vi "PCO_Init.vi"() -> (0 "ErrorOut":errorcluster, 2 "BufferID":i16[](array[numeric]), 3 "hout":u64, 4 "SizeVer":u16, 5 "Bits/pixel":u16, 6 "SizeHor":u16, 8 "PixelRates":u32[](array[numeric]))   [LabVIEW 2014]
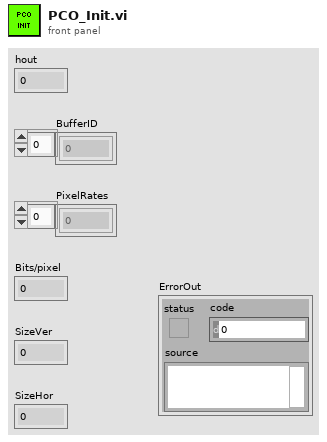
[diagram p1: front panel]
types:
  T1 = cluster{"Size":u16, "SensorTypeDESC":u16, "SensorSubtypeDESC":u16, "MaxHorizontalResStdDESC":u16, "MaxVerticalResStdDESC":u16, "MaxHorizontalResExtDESC":u16, "MaxVerticalResExtDESC":u16, "DynResDESC":u16, "MaxBinHorzDESC":u16, "BinHorzStepDESC":bool, "MaxBinVertDESC":u16, "BinVertStepDESC":bool, "ROIHorzStepDESC":u16, "ROIVertStepDESC":u16, "NumADCDESC":u16, "IRDESC":bool, "MinDelayDESC":u32, "MaxDelayDESC":u32, "MinDelayStepDESC":u32, "MinExpoDESC":u32, "MaxExpoDESC":u32, "MinExpoStepDESC":u32, "MinDelayIRDESC":u32, "MaxDelayIRDESC":u32, "MinExpoIRDESC":u32, "MaxExpoIRDESC":u32, "TimeTableDESC":bool, "DoubleImageDESC":bool, "MinCoolSetDESC":i16, "MaxCoolSetDESC":i16, "MDefaultCoolSetDESC":i16, "PowerDownModeDESC":bool, "OffsetRegDESC":bool, "ColorPattern":cluster{"UpperLeftColor":u8, "UpperRightColor":u8, "LowerLeftColor":u8, "LowerRightColor":u8}, "PatternTypeDESC":bool, "PixelRates":u32[], "CoversionFactors":u16[], "Reserved":u32[], "NoiseFilterCapable":bool, "HotPixelCapable":bool, "HotPixelWithNoiseFilter":bool, "ASCIITimeCapable":bool, "Extended Description":bool, "Get Extended":bool, "Reserved Flag 1":bool, "Reserved Flag 2":bool}
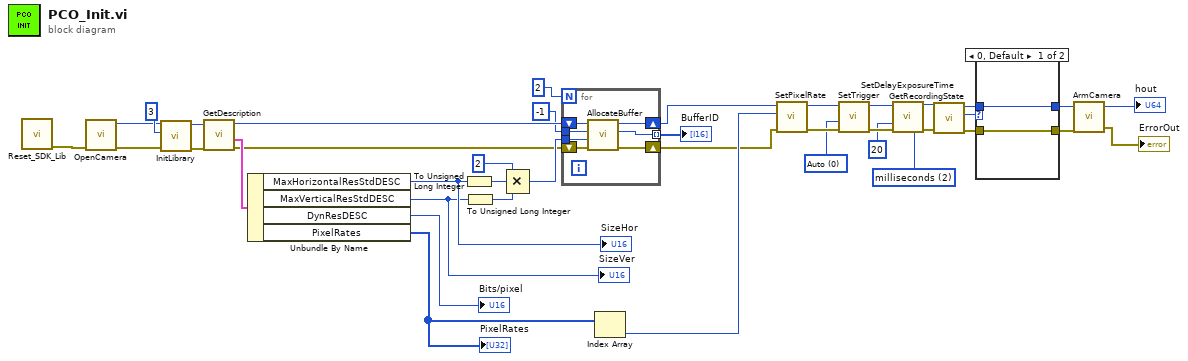
[diagram p0: block diagram]
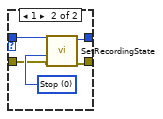
[diagram p2: hidden frame]
diagram:
  w15 = u16 2 items=["nanoseconds", "microseconds", "milliseconds"] ("DelayTimeBase")
  w20 = u16 0 items=["Auto", "Software", "External sequence start ", "External exposure control"] ("TriggerMode")
  n1 = call "Reset_SDK_Lib.vi"() -> ("ErrorOut"=w5:errorcluster)  [unwired: 11 in]
  n2 = call "OpenCamera.vi"("ErrorIn"=w5) -> ("ErrorOut"=w2:errorcluster, "Handle out"=w4:u64)  [unwired: 3 in, 2 out]
  n3 = call "InitLibrary.vi"("error in (no error)"=w2, "InterfaceType"=u32 3, "ph"=w4) -> ("error out"=w1:errorcluster, "hout"=w3:u64)  [unwired: 7 in]
  n4 = call "GetDescription.vi"("ErrorIn"=w1, "ph"=w3) -> ("ErrorOut"=w27:errorcluster, "Description"=w39:T1, "hout"=w38:u64)  [unwired: 2 in, 1 out]
  n5 = Unbundle By Name(w39) -> ("MaxHorizontalResStdDESC"=w29:u16, "MaxVerticalResStdDESC"=w28:u16, "DynResDESC"=→"Bits/pixel":u16, "PixelRates"=w24:u32[])
  "PixelRates" <- w24
  "SizeHor" <- w29
  "SizeVer" <- w28
  n6 = To Unsigned Long Integer(number=w29) -> (unsigned 32bit integer=w32:u32)
  n7 = To Unsigned Long Integer(number=w28) -> (unsigned 32bit integer=w31:u32)
  n8 = Compound Arithmetic op=MULTIPLY(u32 2 ("value"), w32, w31) -> (w33:u32)
  n9 = for {
    N: 2 -> [_]
    shift-right: [w45] -> w26
    shift-left: w38 -> [w46]
    tunnel: i16 -1 ("BufNr") -> [w44]
    tunnel: [w43] -> w35 mode=indexing
    tunnel: w33 -> [w42]
    shift-right: [w40] -> w22
    shift-left: w27 -> [w41]
    n10 = call "AllocateBuffer.vi"("error in (no error)"=w41, "Size"=w42, "BufNr"=w44, "ph"=w46) -> ("error out"=w40:errorcluster, "BufNrOut"=w43:i16, "hout"=w45:u64)  [unwired: 2 in, 3 out]
  }
  "BufferID" <- w35
  n11 = Index Array(array=w24) -> (element=w23:u32)  [unwired: 1 in]
  n12 = call "SetPixelRate.vi"("error in (no error)"=w22, "PixelRate"=w23, "ph"=w26) -> ("error out"=w21:errorcluster, "hout"=w25:u64)  [unwired: 2 in, 1 out]
  n13 = call "SetTrigger.vi"("error in (no error)"=w21, "TriggerMode"=w20, "ph"=w25) -> ("error out"=w18:errorcluster, "hout"=w19:u64)  [unwired: 2 in, 1 out]
  n14 = call "SetDelayExposureTime.vi"("ph"=w19, "Exposure"=u32 20, "error in (no error)"=w18, "ExposureTimeBase"=w15) -> ("hout"=w10:u64, "error out"=w9:errorcluster)  [unwired: 9 in, 1 out]
  n15 = call "GetRecordingState.vi"("ErrorIn"=w9, "ph"=w10) -> ("ErrorOut"=w13:errorcluster, "RecordingState"=w11:u16, "hout"=w12:u64)  [unwired: 2 in, 1 out]
  n16 = case shown="0, Default" w11 {
    tunnel: w12 -> [w48 w52]
    tunnel: w13 -> [w47 w51]
    tunnel: [w48 w50] -> w8
    tunnel: [w47 w49] -> w7
    frame 0, Default {
    }
    frame 1 {
      w53 = u16 0 items=["Stop", "Run"] ("RecordingState")
      n17 = call "SetRecordingState.vi"("ErrorIn"=w51, "RecordingState"=w53, "ph"=w52) -> ("ErrorOut"=w49:errorcluster, "hout"=w50:u64)  [unwired: 2 in, 1 out]
    }
  }
  n18 = call "ArmCamera.vi"("error in (no error)"=w7, "ph"=w8) -> ("error out"=→"ErrorOut":errorcluster, "hout"=→"hout":u64)  [unwired: 1 in, 1 out]
